vi "norma4000_daq.vi"() -> ()   [LabVIEW 2020]
panel:
  out "Loop Rate (Hz)":u32
  in  "Instrument Descriptor (ASRL1::INSTR)":string="ASRL1::INSTR"
  out "Saving In Progress":bool
  in  "file path":path
  out "Error Message (empty)":string
  out "Error Code (0)":i32 format="%.0x"
  in  "STOP":bool=TRUE
  # "TCPIP0::192.168.0.103::23::SOCKET"
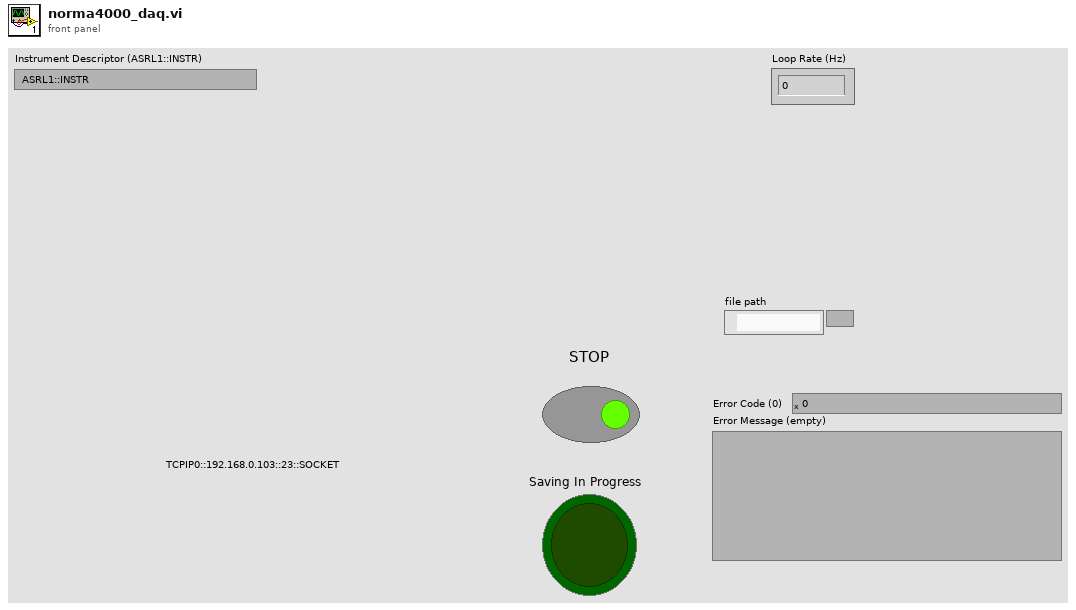
[diagram p1: front panel]
types:
  T1 = enum16{"open", "open or create", "create or replace", "create", "open (read-only)"}
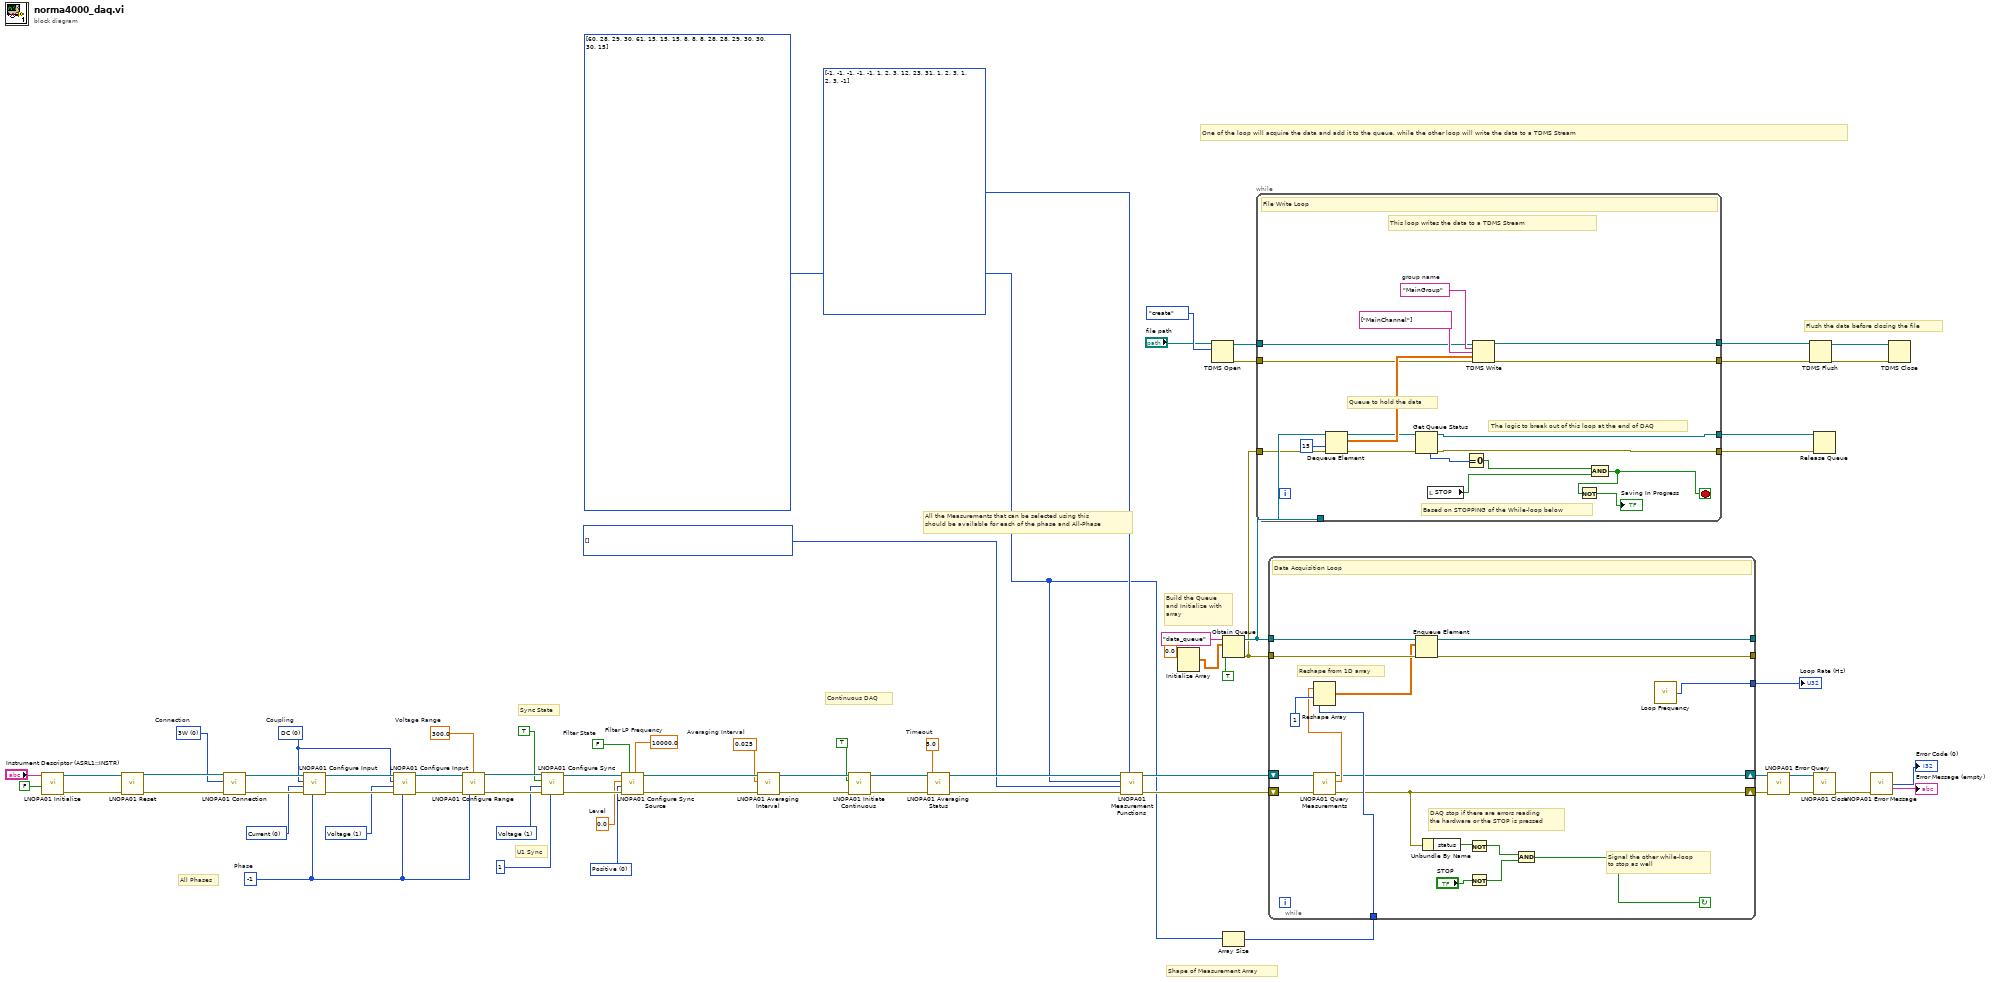
[diagram p0: block diagram]
diagram:
  w7 = i32[] [] items=["None", "Minimum", "Maximum", "Integral Positive", "Integral Negative", "Integral"] ("Modifier")
  w8 = i32[] [60, 28, 29, 30, 61, 15, 15, 15, 8, 8, 8, 28, 28, 29, 30, 30, 30, 15] items=["Voltage True RMS", "Voltage Mean", "Voltage Rectified Mean ", "Voltage Peak-To-Peak ", "Voltage Highest Value ", "Voltage Lowest Value ", "Voltage Crest Factor", "Voltage Absolute Phase", "Voltage True RMS Phase-To-Phase", "Voltage Harmonic", "Voltage TRMS Phase-To-Phase Harmonic", "Voltage Form Factor", "Voltage Harmonic Content", "Voltage Fundamental Content", "Voltage THD", "Current True RMS", "Current Mean", "Current Rectified Mean ", "Current Peak-To-Peak ", "Current Highest Value ", "Current Lowest Value", "Current Crest Factor", "Current Absolute Phase", "Current Harmonic", "Current Form Factor", "Current Harmonic Content", "Current Fundamental Content", "Current THD", "Power Active", "Power Apparent", "Power Reactive", "Power Factor", "Power Active Harmonic", "Power Apparent Harmonic", "Power Reactive Harmonic", "Power Factor Harmonic", "Power Corrected", "Phase", "Phase Harmonic", "Impedance", "Resistance Serial", "Resistance Parallel", "Reactance Serial", "Reactance Parallel", "Impedance Harmonic", "Resistance Serial Harmonic", "Resistance Parallel Harmonic", "Reactance Serial Harmonic", "Reactance Parallel Harmonic", "Frequency", "Averaging Interval", "Shaft Torque", "Rotational Speed", "Mechanical Power", "Rotational Asynchronousity", "Motor Efficiency", "Raw Process Input Value ", "Voltage Mean Phase-To-Phase", "Voltage Rectified Mean Phase-To-Phase", "Voltage Form Factor Phase-To-Phase", "Averaging Interval Relative Timestamp", "Electrical Efficiency", "Electrical Efficiency Harmonic", "True RMS Voltage Without DC", "True RMS Current Without DC", "Voltage THD Phase-To-Phase", "Voltage Harmonic Content Phase-To-Phase", "Voltage Fundamental Content Phase-To-Phase", "Voltage Rectified Mean Corrected", "Voltage Rectified Mean Phase-To-Phase Corrected", "Current Rectified Mean Corrected"] ("Measurement")
  w37 = 5.0  # Timeout
  w43 = 0.025  # Averaging Interval
  w46 = 0 items=["Positive", "Negative"] ("Slope")
  w47 = 0.0  # Level
  w48 = 10000.0  # Filter LP Frequency
  w49 = FALSE  # Filter State
  w53 = 1 items=["Current", "Voltage", "External"] ("Channel")
  w57 = 300.0  # Voltage Range
  w61 = 1 items=["Current", "Voltage"] ("Channel")
  w58 = -1  # Phase
  w65 = 0 items=["Current", "Voltage"] ("Channel")
  w62 = 0 items=["DC", "AC"]  # Coupling
  w68 = 0 items=["3W", "2W"]  # Connection
  # "All the Measurements that can be selected using this\nshould be available for each of the phase and All-Phase"
  # "Build the Queue\nand Initialize with\narray"
  # "Flush the data before closing the file"
  # "One of the loop will acquire the data and add it to the queue, while the other loop will write the data to a TDMS Stream"
  # "Shape of Measurement Array"
  # "Continuous DAQ"
  # "U1 Sync"
  # "Sync State"
  # "All Phases"
  n1 = call <instrlib>:"LNOPA01 Initialize.vi"("Reset (T: Reset)"=FALSE, "Instrument Descriptor (ASRL1::INSTR)"="Instrument Descriptor (ASRL1::INSTR)") -> ("error out"=w3:errorcluster, "VISA session"=w4:refnum<visa-resource-name>)  [unwired: 8 in]
  n2 = call <instrlib>:"LNOPA01 Reset.vi"("VISA session"=w4, "error in (no error)"=w3) -> ("dup VISA session"=w70:refnum<visa-resource-name>, "error out"=w69:errorcluster)  [unwired: 12 in]
  n3 = call <instrlib>:"LNOPA01 Connection.vi"("error in (no error)"=w69, "Connection"=w68, "VISA session"=w70) -> ("error out"=w67:errorcluster, "dup VISA session"=w66:refnum<visa-resource-name>)  [unwired: 6 in, 1 out]
  n4 = call <instrlib>:"LNOPA01 Configure Input.vi"("Phase"=w58, "error in (no error)"=w67, "Channel"=w65, "Coupling"=w62, "VISA session"=w66) -> ("error out"=w63:errorcluster, "dup VISA session"=w64:refnum<visa-resource-name>)  [unwired: 5 in]
  n5 = call <instrlib>:"LNOPA01 Configure Input.vi"("Phase"=w58, "error in (no error)"=w63, "Channel"=w61, "Coupling"=w62, "VISA session"=w64) -> ("error out"=w59:errorcluster, "dup VISA session"=w60:refnum<visa-resource-name>)  [unwired: 5 in]
  n6 = call <instrlib>:"LNOPA01 Configure Range.vi"("VISA session"=w60, "Voltage Range"=w57, "error in (no error)"=w59, "Phase"=w58) -> ("dup VISA session"=w56:refnum<visa-resource-name>, "error out"=w55:errorcluster)  [unwired: 10 in]
  n7 = call <instrlib>:"LNOPA01 Configure Sync.vi"("Phase"=1, "error in (no error)"=w55, "Channel"=w53, "State"=TRUE, "VISA session"=w56) -> ("error out"=w50:errorcluster, "dup VISA session"=w51:refnum<visa-resource-name>)  [unwired: 5 in]
  n8 = call <instrlib>:"LNOPA01 Configure Sync Source.vi"("Filter LP Frequency"=w48, "Filter State"=w49, "error in (no error)"=w50, "Slope"=w46, "Level"=w47, "VISA session"=w51) -> ("error out"=w44:errorcluster, "dup VISA session"=w45:refnum<visa-resource-name>)  [unwired: 4 in]
  n9 = call <instrlib>:"LNOPA01 Averaging Interval.vi"("error in (no error)"=w44, "Averaging Interval"=w43, "VISA session"=w45) -> ("error out"=w41:errorcluster, "dup VISA session"=w42:refnum<visa-resource-name>)  [unwired: 6 in, 1 out]
  n10 = call <instrlib>:"LNOPA01 Initiate Continuous.vi"("error in (no error)"=w41, "State"=TRUE, "VISA session"=w42) -> ("error out"=w38:errorcluster, "dup VISA session"=w39:refnum<visa-resource-name>)  [unwired: 6 in, 1 out]
  n11 = call <instrlib>:"LNOPA01 Averaging Status.vi"("error in (no error)"=w38, "Timeout"=w37, "VISA session"=w39) -> ("error out"=w35:errorcluster, "dup VISA session"=w36:refnum<visa-resource-name>)  [unwired: 6 in, 1 out]
  n12 = call <instrlib>:"LNOPA01 Measurement Functions.vi"("Phase"=i32[] [-1, -1, -1, -1, -1, 1, 2, 3, 12, 23, 31, 1, 2, 3, 1, 2, 3, -1], "error in (no error)"=w35, "Modifier"=w7, "Measurement"=w8, "VISA session"=w36) -> ("error out"=w33:errorcluster, "dup VISA session"=w34:refnum<visa-resource-name>)  [unwired: 2 in, 3 out]
  n13 = Initialize Array(0.0 ("element")) -> (w21:dbl[][])  [unwired: 2 in]
  n14 = TDMS Open(10:T1."create" ("operation (0:open)"), 11:"file path") -> (0:w11:errorcluster, 3:w10:refnum<k34>)  [unwired: 5 in]
  n15 = Obtain Queue(name (unnamed)="data_queue", element data type=w21, create if not found? (T)=TRUE) -> (queue out=w23:refnum<queue>, error out=w22:errorcluster)  [unwired: 2 in, 1 out]
  n16 = Array Size(array=w8) -> (size(s)=w19:i32)
  n17 = while {
    tunnel: w23 -> [w87]
    tunnel: w22 -> [w86]
    tunnel: [w81] -> w18
    tunnel: [w73] -> w17
    tunnel: [w80] -> w14
    tunnel: [w79] -> w13
    tunnel: w11 -> [w78]
    tunnel: w10 -> [w77]
    stop <- w72 stop-if-true
    w89 = "MainGroup"  # group name
    # "Based on STOPPING of the While-loop below"
    # "Queue to hold the data"
    # "The logic to break out of this loop at the end of DAQ"
    # "This loop writes the data to a TDMS Stream"
    # "File Write Loop"
    n18 = Dequeue Element(queue=w87, timeout in ms (-1)=15, error in (no error)=w86) -> (queue out=w84:refnum<queue>, element=w85:dbl[][], error out=w83:errorcluster)  [unwired: 1 out]
    n19 = Get Queue Status(queue=w84, error in (no error)=w83) -> (queue out=w80:refnum<queue>, error out=w79:errorcluster, # elements in queue=w82:i32)  [unwired: 1 in, 5 out]
    n20 = local read "STOP"() -> (w74:bool)
    n21 = Equal To 0?(x=w82) -> (x = 0?=w76:bool)
    n22 = TDMS Write(0:w77, 5:w89, 7:string[] ["MainChannel"] ("channel name(s) in (Untitled)"), 9:w85, 11:w78) -> (4:w81:refnum<k34>, 15:w73:errorcluster)  [unwired: 1 in, 2 out]
    n23 = And(x=w76, y=w74) -> (x .and. y?=w72:bool)
    n24 = Not(x=w72) -> (.not. x?=→"Saving In Progress":bool)
  }
  n25 = while {
    tunnel: w19 -> [w103]
    shift-right: [w98] -> w32
    shift-left: w34 -> [w107]
    shift-right: [w102] -> w31
    shift-left: w33 -> [w106]
    tunnel: w23 -> [w97]
    tunnel: w22 -> [w96]
    tunnel: [w95] -> _
    tunnel: [w94] -> _
    tunnel: [w90] -> w1
    stop <- w93 continue-if-true
    # "Reshape from 1D array"
    # "Signal the other while-loop\nto stop as well"
    # "DAQ stop if there are errors reading\nthe hardware or the STOP is pressed"
    # "Data Acquisition Loop"
    n26 = call <instrlib>:"LNOPA01 Query Measurements.vi"("error in (no error)"=w106, "VISA session"=w107) -> ("error out"=w102:errorcluster, "Data"=w104:dbl[], "dup VISA session"=w98:refnum<visa-resource-name>)  [unwired: 7 in]
    n27 = Reshape Array(w104, 1 ("dimension size"), w103) -> (w91:dbl[][])
    n28 = Enqueue Element(queue=w97, element=w91, error in (no error)=w96) -> (queue out=w95:refnum<queue>, error out=w94:errorcluster)  [unwired: 1 in, 1 out]
    n29 = Unbundle By Name(w102) -> ("status"=w101:bool)
    n30 = Not(x=w101) -> (.not. x?=w100:bool)
    n31 = Not(x="STOP") -> (.not. x?=w99:bool)
    n32 = And(x=w100, y=w99) -> (x .and. y?=w93:bool)
    n33 = call "Loop Frequency.vi"() -> ("Loop Rate (Hz)"=w90:u32)
  }
  "Loop Rate (Hz)" <- w1
  n34 = call <instrlib>:"LNOPA01 Error Query.vi"("error in (no error)"=w31, "VISA session"=w32) -> ("error out"=w29:errorcluster, "dup VISA session"=w30:refnum<visa-resource-name>)  [unwired: 6 in, 2 out]
  n35 = TDMS Flush(4:w17, 7:w18) -> (0:w15:errorcluster, 3:w16:refnum<k34>)
  n36 = Release Queue(queue=w14, error in (no error)=w13) -> ()  [unwired: 1 in, 3 out]
  n37 = call <instrlib>:"LNOPA01 Close.vi"("error in (no error)"=w29, "VISA session"=w30) -> ("error out"=w24:errorcluster)  [unwired: 9 in]
  n38 = call <instrlib>:"LNOPA01 Error Message.vi"("error in (no error)"=w24) -> ("Error Code (0)"=→"Error Code (0)":i32, "Error Message (empty)"=→"Error Message (empty)":string)  [unwired: 10 in, 3 out]
  n39 = TDMS Close(8:w15, 11:w16) -> ()  [unwired: 2 out]
